vi "Interface_Dispatch_Get Parameter Control Refs.vi"(8 "error in (no error)":errorcluster, 11 "Dispatch_Demand Limiting in":refnum<class "Dispatch_Demand Limiting.lvclass">) -> (0 "error out":errorcluster, 1 "Output Controls[]":refnum<vi>[](array[refnum]), 2 "Configuration Controls[]":refnum<vi>[](array[refnum]), 3 "Dispatch_Demand Limiting out":refnum<class "Dispatch_Demand Limiting.lvclass">, 4 "Dependencies Controls[]":refnum<vi>[](array[refnum]))   [LabVIEW 2015, in "Dispatch_Demand Limiting.lvclass"]
uses:
  Dispatch_Demand Limiting.lvclass
  Dispatch_Demand Limiting_Configuration.ctl
  Dispatch_Demand Limiting_Dependencies.ctl
  Dispatch_Demand Limiting_Output.ctl
  Dispatch_Demand Limiting.lvclass/Dispatch_Demand Limiting.ctl
panel:
  out "Output":T1
  out "Dependencies":T2
  out "Configuration":T3
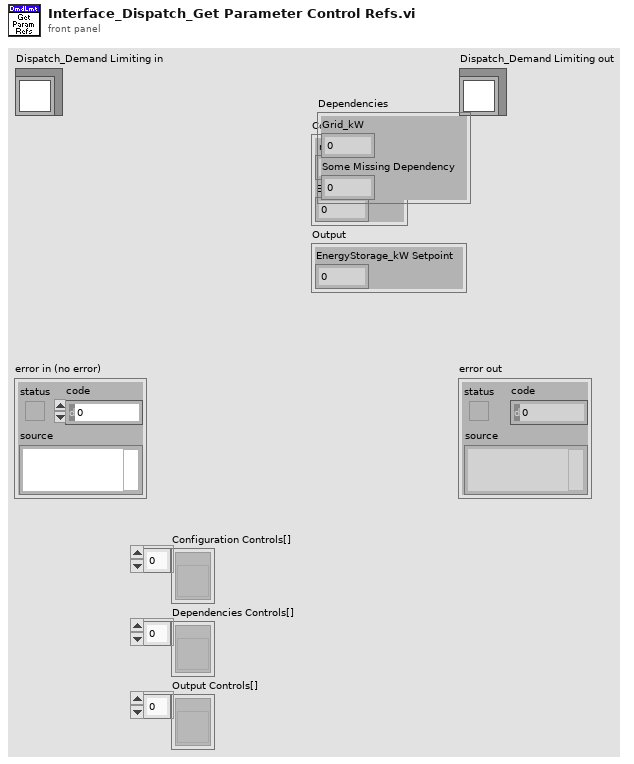
[diagram p1: front panel]
types:
  T1 = typedef "Dispatch_Demand Limiting.lvclass/Dispatch_Demand Limiting_Output.ctl" = cluster{"EnergyStorage_kW Setpoint":dbl}
  T2 = typedef "Dispatch_Demand Limiting.lvclass/Dispatch_Demand Limiting_Dependencies.ctl" = cluster{"Grid_kW":dbl, "Some Missing Dependency":dbl}
  T3 = typedef "Dispatch_Demand Limiting.lvclass/Dispatch_Demand Limiting_Configuration.ctl" = cluster{"Import kW Limit":dbl, "Export kW Limit":dbl}
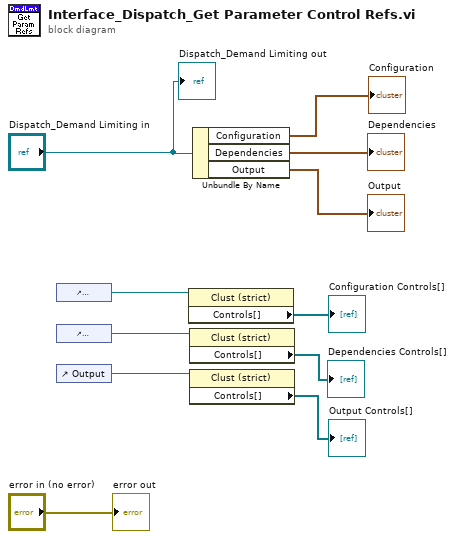
[diagram p0: block diagram]
diagram:
  n1 = control-ref of="Configuration"() -> (w5:refnum<vi>)
  n2 = control-ref of="Dependencies"() -> (w3:refnum<vi>)
  n3 = control-ref of="Output"() -> (w4:refnum<vi>)
  n4 = property class="Clust (strict)"(reference=w5) -> ("Controls[]"=→"Configuration Controls[]":refnum<vi>[])  [unwired: 1 in, 2 out]
  n5 = property class="Clust (strict)"(reference=w3) -> ("Controls[]"=→"Dependencies Controls[]":refnum<vi>[])  [unwired: 1 in, 2 out]
  n6 = property class="Clust (strict)"(reference=w4) -> ("Controls[]"=→"Output Controls[]":refnum<vi>[])  [unwired: 1 in, 2 out]
  n7 = Unbundle By Name("Dispatch_Demand Limiting in") -> ("Configuration"=→"Configuration":T3, "Dependencies"=→"Dependencies":T2, "Output"=→"Output":T1)
  "error out" <- "error in (no error)"
  "Dispatch_Demand Limiting out" <- "Dispatch_Demand Limiting in"
